vi "Line2003.vi"   [LabVIEW 2013]
uses:
  <vilib>/Heliosphere Research LLC/Advanced Plotting Toolkit/Advanced Plotting Toolkit.lvlib
types:
  T1 = typedef "Advanced Plotting Toolkit.lvlib/PlotID.ctl" = i32
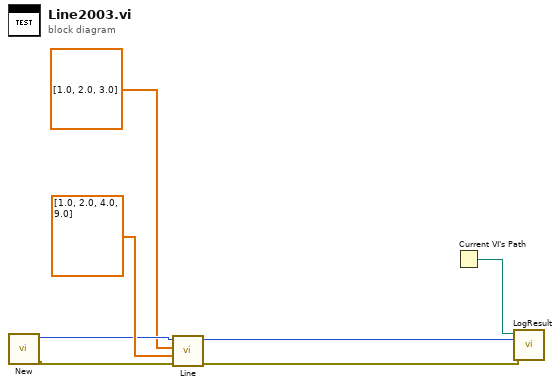
[diagram p0: block diagram]
diagram:
  n1 = call <vilib>:"New.vi"() -> ("error out"=w3:errorcluster, "Plot ID"=w5:T1)  [unwired: 10 in]
  n2 = call <vilib>:"Line.vi"("error in (no error)"=w3, "Y Data"=dbl[] [1.0, 2.0, 4.0, 9.0], "X Data"=dbl[] [1.0, 2.0, 3.0], "Plot ID"=w5) -> ("error out"=w2:errorcluster, "Plot ID out"=w4:T1)  [unwired: 6 in]
  n3 = Current VI's Path() -> (path=w7:path)
  n4 = call "LogResult.vi"("Test Result"=w2, "Test Artifact"=w4, "VI Path"=w7) -> ()  [unwired: 9 in]
